vi "Move Stage.vi"(8 "error in (no error)":errorcluster, 11 "Input Coor":cluster{"X":sgl, "Y":sgl}) -> (0 "error out":errorcluster)   [LabVIEW 2017]
doc: "Use this template to build a VI to use as a subVI."
uses:
  AEROTECstageAPI/StageEnum.ctl
  AEROTECstageAPI/MoveDistanceInAxis.ctl
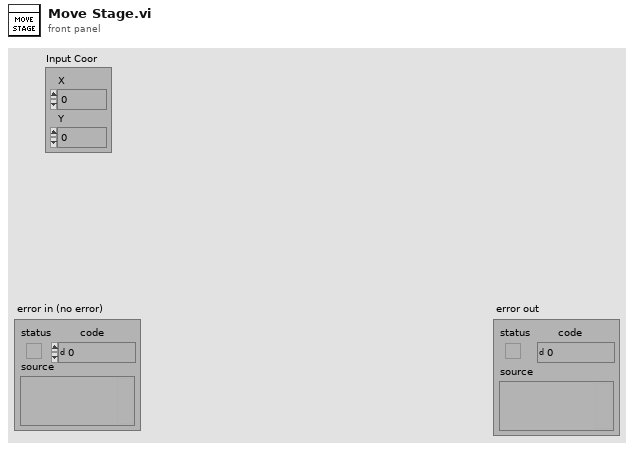
[diagram p1: front panel]
types:
  T1 = typedef "StageEnum.ctl" = enum16{"Get Current Pos!", "Move axis!", "Enable Stage!", "Stop Stage Controller!", "Set Default Speeds!", "Get Stage Parameters", "Start Stage Controller!", "Init", "Go Home!"}
  T2 = typedef "MoveDistanceInAxis.ctl" = cluster{"Axis Number":i16, "Distance (microns)":dbl}
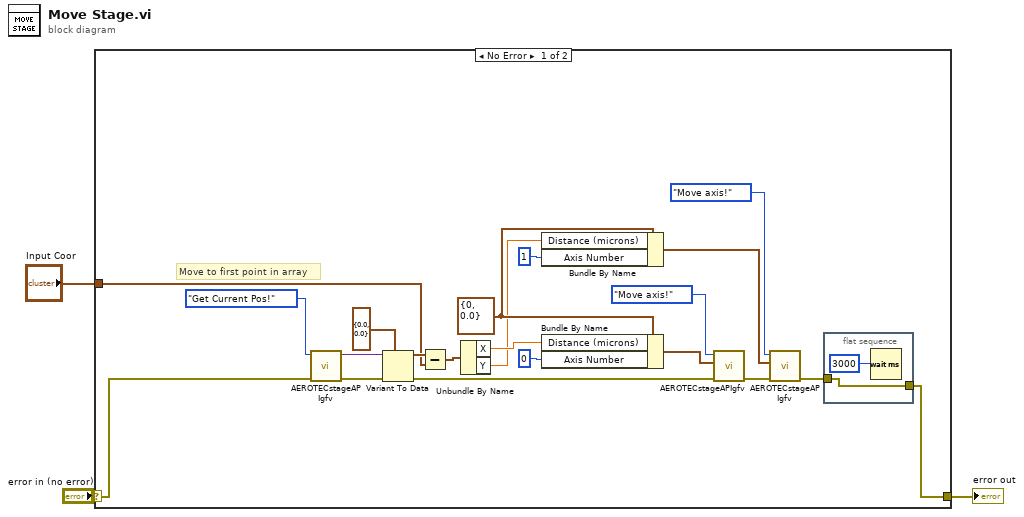
[diagram p0: block diagram]
diagram:
  n1 = case shown="No Error" "error in (no error)" {
    selector: "error in (no error)" -> [w7 w27]
    tunnel: [w4 w27] -> w2
    tunnel: "Input Coor" -> [w6 _]
    frame No Error {
      w10 = T2 {"Axis Number"=0, "Distance (microns)"=0.0} ("MoveDistanceInAxis")
      # "Move to first point in array"
      n2 = call "AEROTECstageAPIgfv.vi"("error in (no error)"=w7, "StageContrlEnum"=StageEnum."Get Current Pos!") -> ("error out"=w21:errorcluster, "Data Out"=w23:variant)  [unwired: 8 in]
      n3 = Variant To Data(error in=w21, type=cluster{"X":sgl, "Y":sgl} {"X"=0.0, "Y"=0.0}, Variant=w23) -> (data=w8:cluster{"X":sgl, "Y":sgl}, error out=w19:errorcluster)
      n4 = Subtract(x=w8, y=w6) -> (x-y=w20:cluster{"X":sgl, "Y":sgl})
      n5 = Unbundle By Name(w20) -> ("X"=w17:sgl, "Y"=w9:sgl)
      n6 = Bundle By Name(cluster=w10, "Distance (microns)"=w9, "Axis Number"=i16 1) -> (w14:T2)
      n7 = Bundle By Name(cluster=w10, "Distance (microns)"=w17, "Axis Number"=i16 0) -> (w15:T2)
      n8 = call "AEROTECstageAPIgfv.vi"("error in (no error)"=w19, "Data in"=w15, "StageContrlEnum"=StageEnum."Move axis!") -> ("error out"=w11:errorcluster)  [unwired: 7 in, 1 out]
      n9 = call "AEROTECstageAPIgfv.vi"("error in (no error)"=w11, "Data in"=w14, "StageContrlEnum"=StageEnum."Move axis!") -> ("error out"=w5:errorcluster)  [unwired: 7 in, 1 out]
      n10 = flat-sequence {
        tunnel: w5 -> [w25]
        tunnel: [w25] -> w4
        frame #0 {
          n11 = Wait (ms)(milliseconds to wait=u32 3000) -> ()  [unwired: 1 out]
        }
      }
    }
    frame Error {
    }
  }
  "error out" <- w2
